vi "Global_HW_Status.vi"() -> ()   [LabVIEW 2017, in "Climber.lvlib"]
uses:
  Climber.lvlib
  TypeDefs/Cluster_SRX Status No Encoder.ctl
panel:
  out "HW_Climber_Status":T1
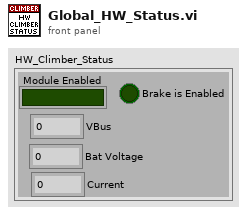
[diagram p1: front panel]
types:
  T1 = typedef "Cluster_SRX Status No Encoder.ctl" = cluster{"VBus ":dbl, "Module Enabled":bool, "Current":dbl, "Brake is Enabled":bool, "Bat Voltage":dbl}
diagram:
